vi "Read Attributes.vi"(11 "Set DER Control Msg":refnum<class "Set DER Control Msg.lvclass">) -> (2 "Payload":cluster{"DER_Control":T1})   [LabVIEW 2018, in "Device Communication and Control Abstract Actor.lvlib" / "Set DER Control Msg.lvclass"]
uses:
  Set DER Control Msg.lvclass
  <vilib>/ORNL/CSEISMIC DDS/CSEISMIC DDS Base/Data Types/DER_Control.ctl
  <vilib>/ORNL/CSEISMIC DDS/CSEISMIC DDS Base/Data Types/Controls/DeviceID.ctl
  Set DER Control Msg.lvclass/Set DER Control Msg.ctl
  <vilib>/ORNL/CSEISMIC DDS/CSEISMIC DDS Base/CSEISMIC DDS.lvclass
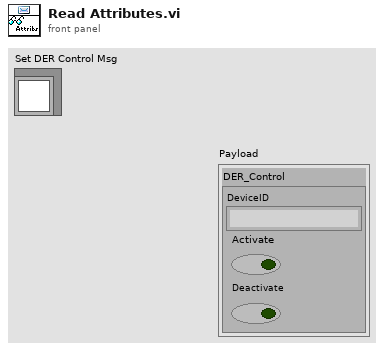
[diagram p1: front panel]
types:
  T1 = typedef "CSEISMIC DDS.lvlib/CSEISMIC DDS.lvclass/DER_Control.ctl" = cluster{"DeviceID":T2, "Activate":bool, "Deactivate":bool}
  T2 = typedef "CSEISMIC DDS.lvlib/CSEISMIC DDS.lvclass/DeviceID.ctl" = string
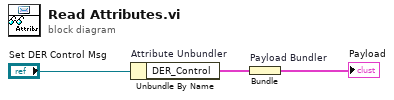
[diagram p0: block diagram]
diagram:
  n1 = Unbundle By Name "Attribute Unbundler"("Set DER Control Msg") -> ("DER_Control"=w1:T1)
  n2 = Bundle "Payload Bundler"("DER_Control"=w1) -> (→"Payload":cluster{"DER_Control":T1})  [unwired: 1 in]
